vi "Generate Error.vi"(4 "Deactive Save Error?":bool, 5 "Actions":T3, 6 "Source":T5, 7 "ErrorData":T2={"Error?"=FALSE, "Error Code"=0, "Classification"=enum."Warning", "Call Chain"=""}, 8 "Error In":errorcluster, 9 "Comment":string, 10 "Description":string, 11 "ErrorLog REF":refnum<class "ErrorLog.lvclass">) -> (0 "Error Out":errorcluster, 3 "Error":refnum<class "Error.lvclass">)   [LabVIEW 2019, in "Error.lvclass"]
uses:
  Error.lvclass
  C:/Projekty/_Wewnetrzne/PC_ActorFramework/07_Program/LABVIEW/02_Source/Classes/EventsAbstract/EventsAbstract.lvclass
  SubModules/LogsAbstract/TypeDef/Event Source.ctl
  EventsAbstract/TypeDef/Event Actions.ctl
  Modules/ModuleAbstract/TypeDef/Module Actions.ctl
  <vilib>/ActorFramework/Message Enqueuer/Message Enqueuer.lvclass
  SubModules/ErrorLog/ErrorLog.lvclass
  TypeDef/Error Classification.ctl
  Error.lvclass/Error.ctl
  EventsAbstract/EventsAbstract.lvclass
  Modules/ModuleAbstract/ModuleAbstract.lvclass
  SubModules/LogsAbstract/LogsAbstract.lvclass
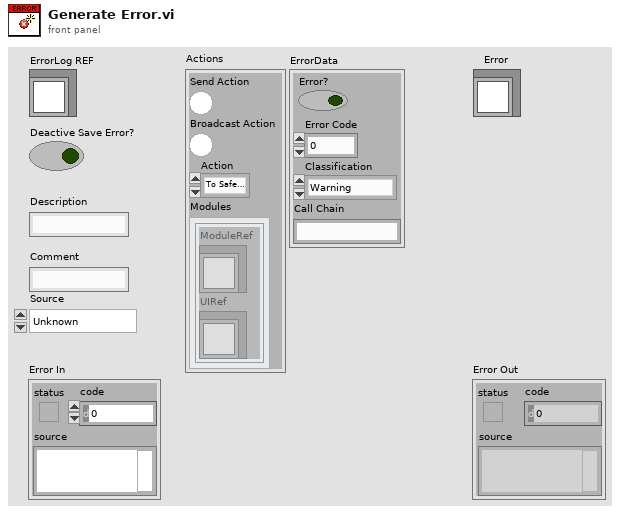
[diagram p1: front panel]
types:
  T1 = typedef "Error.lvclass/Error Classification.ctl" = enum16{"System Error", "Process Error", "Warning", "LabView built-in"}
  T2 = cluster{"Error?":bool, "Error Code":i32, "Classification":T1, "Call Chain":string}
  T3 = typedef "EventsAbstract.lvclass/Event Actions.ctl" = cluster{"Send Action":bool, "Broadcast Action":bool, "Action":T4, "Modules":cluster{"ModuleRef":refnum<class "Message Enqueuer.lvclass">, "UIRef":refnum<class "Message Enqueuer.lvclass">}[]}
  T4 = typedef "ModuleAbstract.lvlib/ModuleAbstract.lvclass/Module Actions.ctl" = enum16{"To Safe State", "Reset Safe State", "Close Module"}
  T5 = typedef "LogsAbstract.lvlib/LogsAbstract.lvclass/Event Source.ctl" = enum16{"Unknown", "< --- Modules --- >", "Core", "< --- SubModules --- >", "EventLog -> Core", "ErrorLog -> Core"}
  T6 = cluster{"Date":string, "Time":string, "Description":string, "Comments":string, "Source":T5}
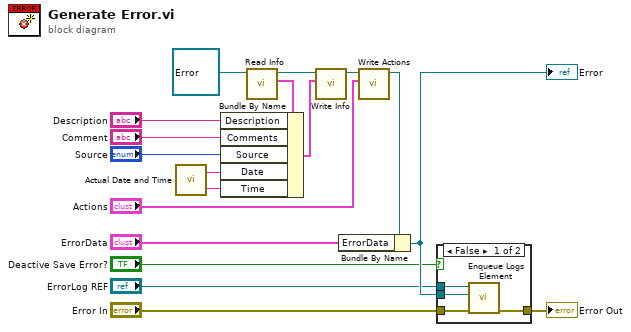
[diagram p0: block diagram]
diagram:
  n1 = call "Actual Date and Time.vi"() -> ("Actual Time"=w7:string, "Actual Date"=w8:string)  [unwired: 2 in]
  n2 = call "Read Info.vi"("EventsAbstract in"=refnum<class "Error.lvclass"> refnum ("Error.lvclass")) -> ("Info"=w5:T6, "EventsAbstract out"=w4:refnum<class "Error.lvclass">)  [unwired: 8 in, 1 out]
  n3 = Bundle By Name(cluster=w5, "Description"="Description", "Comments"="Comment", "Source"="Source", "Date"=w8, "Time"=w7) -> (w3:T6)
  n4 = call "Write Info.vi"("Info"=w3, "EventsAbstract in"=w4) -> ("EventsAbstract out"=w2:refnum<class "Error.lvclass">)  [unwired: 8 in, 1 out]
  n5 = call "Write Actions.vi"("Actions"="Actions", "EventsAbstract in"=w2) -> ("EventsAbstract out"=w1:refnum<class "Error.lvclass">)  [unwired: 8 in, 1 out]
  n6 = Bundle By Name(cluster=w1, "ErrorData"="ErrorData") -> (w12:refnum<class "Error.lvclass">)
  "Error" <- w12
  n7 = case shown="False" "Deactive Save Error?" {
    tunnel: "Error In" -> [w22 w23]
    tunnel: [w21 w23] -> w17
    tunnel: "ErrorLog REF" -> [w20 _]
    tunnel: w12 -> [w19 _]
    frame False {
      n8 = call-dynamic "Enqueue Logs Element.vi"("Error In"=w22, "Event Occured"=w19, "EventLog in"=w20) -> ("Error Out"=w21:errorcluster)  [unwired: 6 in, 2 out]
    }
    frame True {
    }
  }
  "Error Out" <- w17
